vi "XIPIN_LTE_DL_Channel_Encoder_1_0.vi"   [LabVIEW 2017]
doc: "The LTE DL Channel Encoder core provides designers with an LTE Downlink Channel Encoding block for the 3GPP TS 36.212 v8.2.0 Multiplexing and channel coding specification.\n------------------------------------\n<b>Need License</b> : Yes"
uses:
  <vilib>/rvi/XilinxIP/XIPIN_XNode/niFpgaXIPIN.xnode
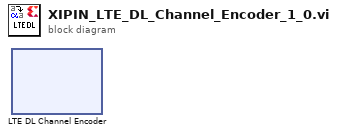
[diagram p0: block diagram]
diagram:
  n1 = xnode ("LTE DL Channel Encoder")() -> ()
